vi "Expand Bounds 1D.vi"(10 "Tolerance (N)":dbl, 11 "Entry":T1[](array[typedef]) {"Axial Force" format="%.4f"; "Lateral Force" format="%.4f"}) -> (2 "Bottom":T1 {"Axial Force" format="%.4f"; "Lateral Force" format="%.4f"}, 3 "Top":T1 {"Axial Force" format="%.4f"; "Lateral Force" format="%.4f"})   [LabVIEW 2016]
uses:
  Typedefs/ForcePair.ctl
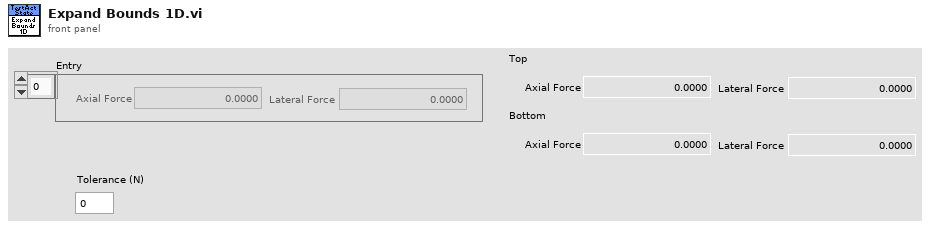
[diagram p1: front panel]
types:
  T1 = typedef "ForcePair.ctl" = cluster{"Axial Force":dbl, "Lateral Force":dbl}
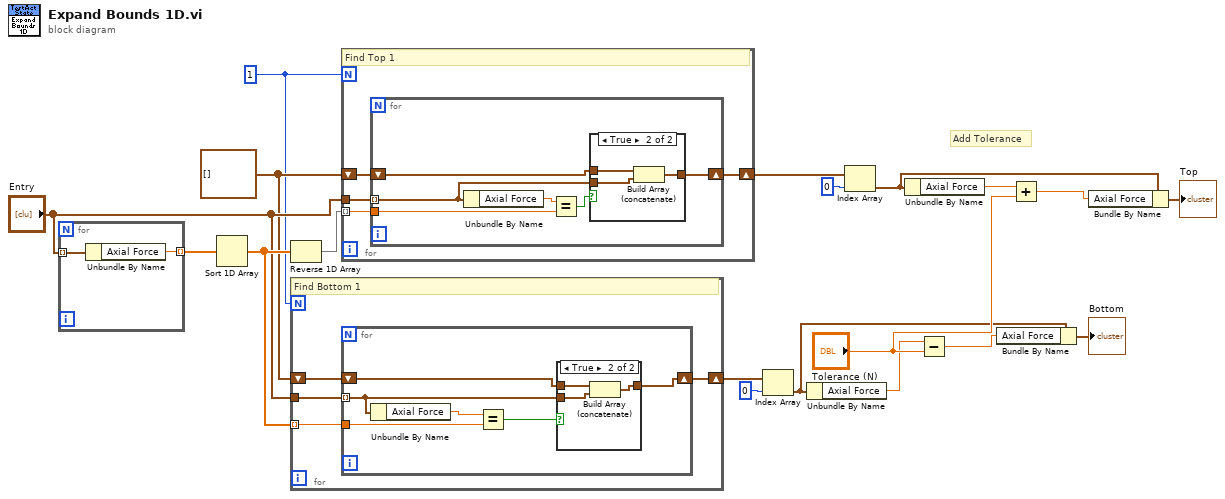
[diagram p0: block diagram]
diagram:
  w15 = T1[] []
  w9 = 1
  # "Add Tolerance"
  n1 = for {
    tunnel: "Entry" -> [w21] mode=indexing
    tunnel: [w20] -> w19 mode=indexing
    n2 = Unbundle By Name(w21) -> ("Axial Force"=w20:dbl)
  }
  n3 = Sort 1D Array(array=w19) -> (sorted array=w17:dbl[])
  n4 = Reverse 1D Array(array=w17) -> (reversed array=w18:dbl[])
  n5 = for {
    N: w9 -> [_]
    tunnel: "Entry" -> [w25]
    tunnel: w17 -> [w22] mode=indexing
    shift-right: [w24] -> w13
    shift-left: w15 -> [w23]
    # "Find Bottom 1"
    n6 = for {
      tunnel: w25 -> [w29] mode=indexing
      shift-right: [w31] -> w24
      shift-left: w23 -> [w30]
      tunnel: w22 -> [w27]
      n7 = Unbundle By Name(w29) -> ("Axial Force"=w28:dbl)
      n8 = Equal?(x=w28, y=w27) -> (x = y?=w26:bool)
      n9 = case shown="True" w26 {
        tunnel: w29 -> [_ w35]
        tunnel: [w32 w34] -> w31
        tunnel: w30 -> [w32 w33]
        frame False {
        }
        frame True {
          n10 = Build Array (concatenate)(w33, w35) -> (w34:T1[])
        }
      }
    }
  }
  n11 = for {
    N: w9 -> [_]
    tunnel: "Entry" -> [w39]
    tunnel: w18 -> [w36] mode=indexing
    shift-right: [w38] -> w11
    shift-left: w15 -> [w37]
    # "Find Top 1"
    n12 = for {
      tunnel: w39 -> [w43] mode=indexing
      shift-right: [w45] -> w38
      shift-left: w37 -> [w44]
      tunnel: w36 -> [w41]
      n13 = Unbundle By Name(w43) -> ("Axial Force"=w42:dbl)
      n14 = Equal?(x=w42, y=w41) -> (x = y?=w40:bool)
      n15 = case shown="True" w40 {
        tunnel: w43 -> [_ w49]
        tunnel: [w46 w48] -> w45
        tunnel: w44 -> [w46 w47]
        frame False {
        }
        frame True {
          n16 = Build Array (concatenate)(w47, w49) -> (w48:T1[])
        }
      }
    }
  }
  n17 = Index Array(array=w13, index=0) -> (element=w4:T1)
  n18 = Unbundle By Name(w4) -> ("Axial Force"=w6:dbl)
  n19 = Index Array(array=w11, index=0) -> (element=w3:T1)
  n20 = Unbundle By Name(w3) -> ("Axial Force"=w8:dbl)
  n21 = Subtract(x=w6, y="Tolerance (N)") -> (x-y=w5:dbl)
  n22 = Bundle By Name(cluster=w4, "Axial Force"=w5) -> (→"Bottom":T1)
  n23 = Add(x=w8, y="Tolerance (N)") -> (x+y=w10:dbl)
  n24 = Bundle By Name(cluster=w3, "Axial Force"=w10) -> (→"Top":T1)
